vi "[ToBeTest] Continuous Complete Measurament RT.vi"() -> ()   [LabVIEW 2014]
uses:
  <vilib>/FPGAPlugInAG/sbRIO-9636/niLvFpga_Open_sbRIO-9636.vi
  <vilib>/rvi/interface/common/dynamic/niFpgaDynamicAddResources.vi
  <vilib>/FPGAPlugInAG/Dynamic/niLvFpga_Reset_Dynamic.vi
  <vilib>/Utility/error.llb/Error Cluster From Error Code.vi
  <vilib>/rvi/errors/niLvFpgaAdjustHostInterfaceError.vi
  <vilib>/rvi/interface/common/niFpgaWaitOnOcc.vi
  <vilib>/FPGAPlugInAG/Dynamic/niLvFpga_Run_Dynamic.vi
  <vilib>/FPGAPlugInAG/Dynamic/niLvFpga_Abort_Dynamic.vi
  <vilib>/FPGAPlugInAG/Dynamic/niLvFpga_Close_Dynamic.vi
  <vilib>/rvi/interface/nirviOpenFPGA/nirviOpenFPGA.xnode
  FPGA Bitfiles/LaserDistanceSen_FPGATarget_N-ParametricDoub_TAOECtWtfmQ.lvbitx
  FPGA Target/Test VIs/N-Parametric Double FFT Mesurament (MAX BIN DETECT) Test.vi
  FPGA Bitfiles/LaserDistanceSen_FPGATarget_N-ParametricDoub_oZd6Q4K0Aos.lvbitx
  FPGA Target/Test VIs/N-Parametric Double FFT Mesurament (MAX BIN DETECT) SLOW Test.vi
  <vilib>/rvi/interface/nirviMethod/nirviMethod.xnode
  <vilib>/rvi/interface/nirviReadWriteControl/nirviReadWriteControl.xnode
  <vilib>/rvi/interface/nirviCloseFPGA/nirviCloseFPGA.xnode
  <vilib>/rvi/errors/niLvFpgaMergeErrorWithErrorCode.vi
  <vilib>/rvi/interface/Simulation/niFpgaSimulationCallBeginRW.vi
  NiFpgaLv.dll
  <vilib>/Analysis/NI_AALBase.lvlib
  <vilib>/FPGAPlugInAG/Dynamic/niLvFpga_ConfigureFifo_Dynamic.vi
  <vilib>/FPGAPlugInAG/Dynamic/niLvFpga_StartFifo_Dynamic.vi
  <vilib>/FPGAPlugInAG/Dynamic/niLvFpga_ReadFifo_Dynamic.vi
panel:
  out "Rel Std Dev":dbl(graph)
  out "Mean distance":dbl(graph)
  in  "init scart":i32=2000
  out "End":bool
  in  "Fixed Measure?":bool
  in  "#signal":i32=3000
  out "Distance moving Rel Standard Deviation":dbl format="%0.7f"
  out "Distance moving mean":dbl format="%0.7f"
  in  "stop":bool
  # "Mean"
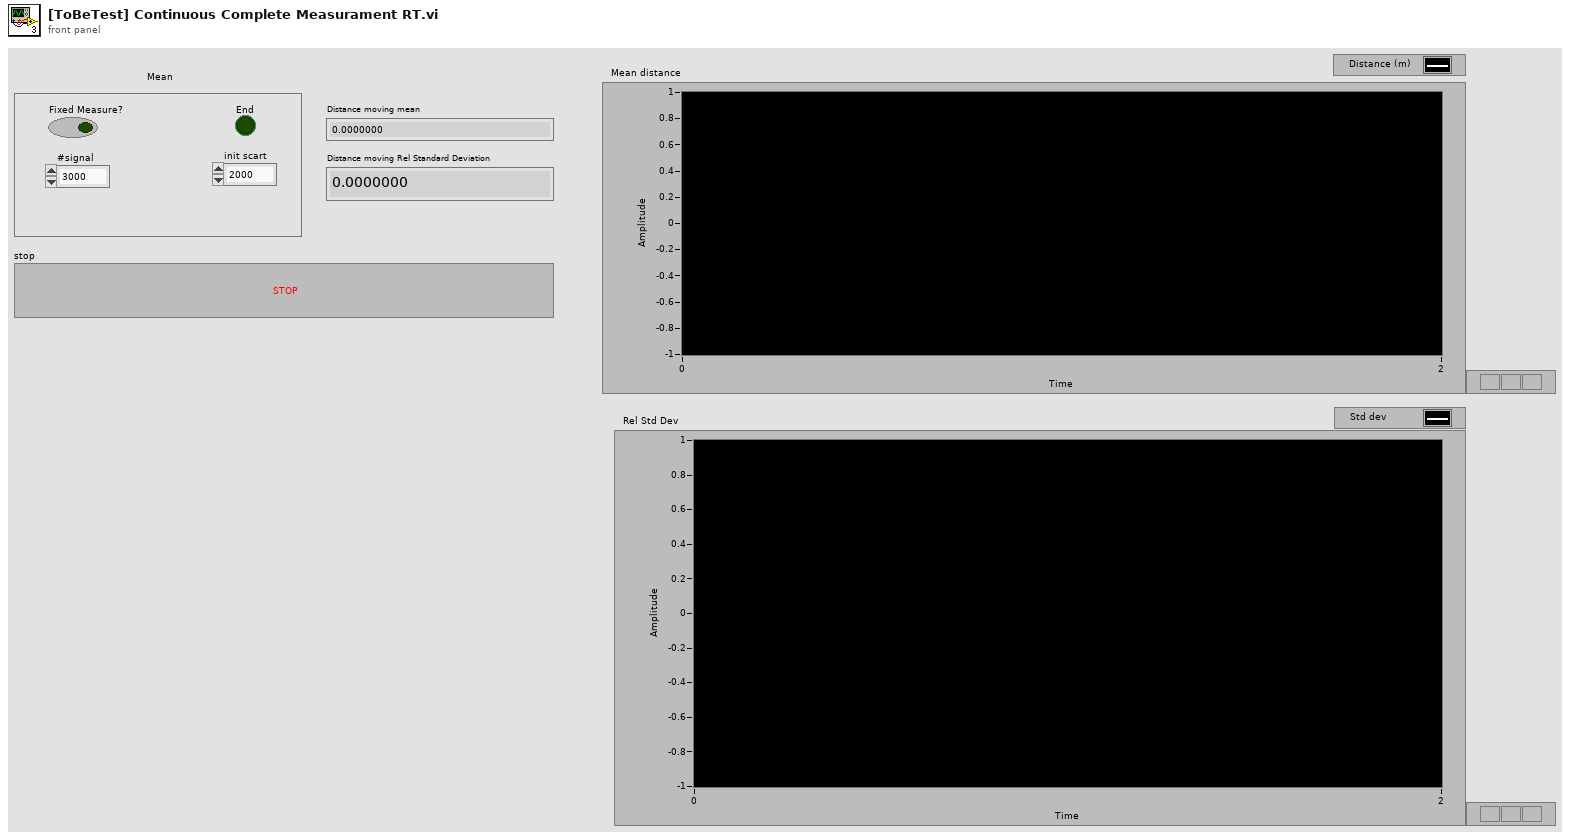
[diagram p1: front panel]
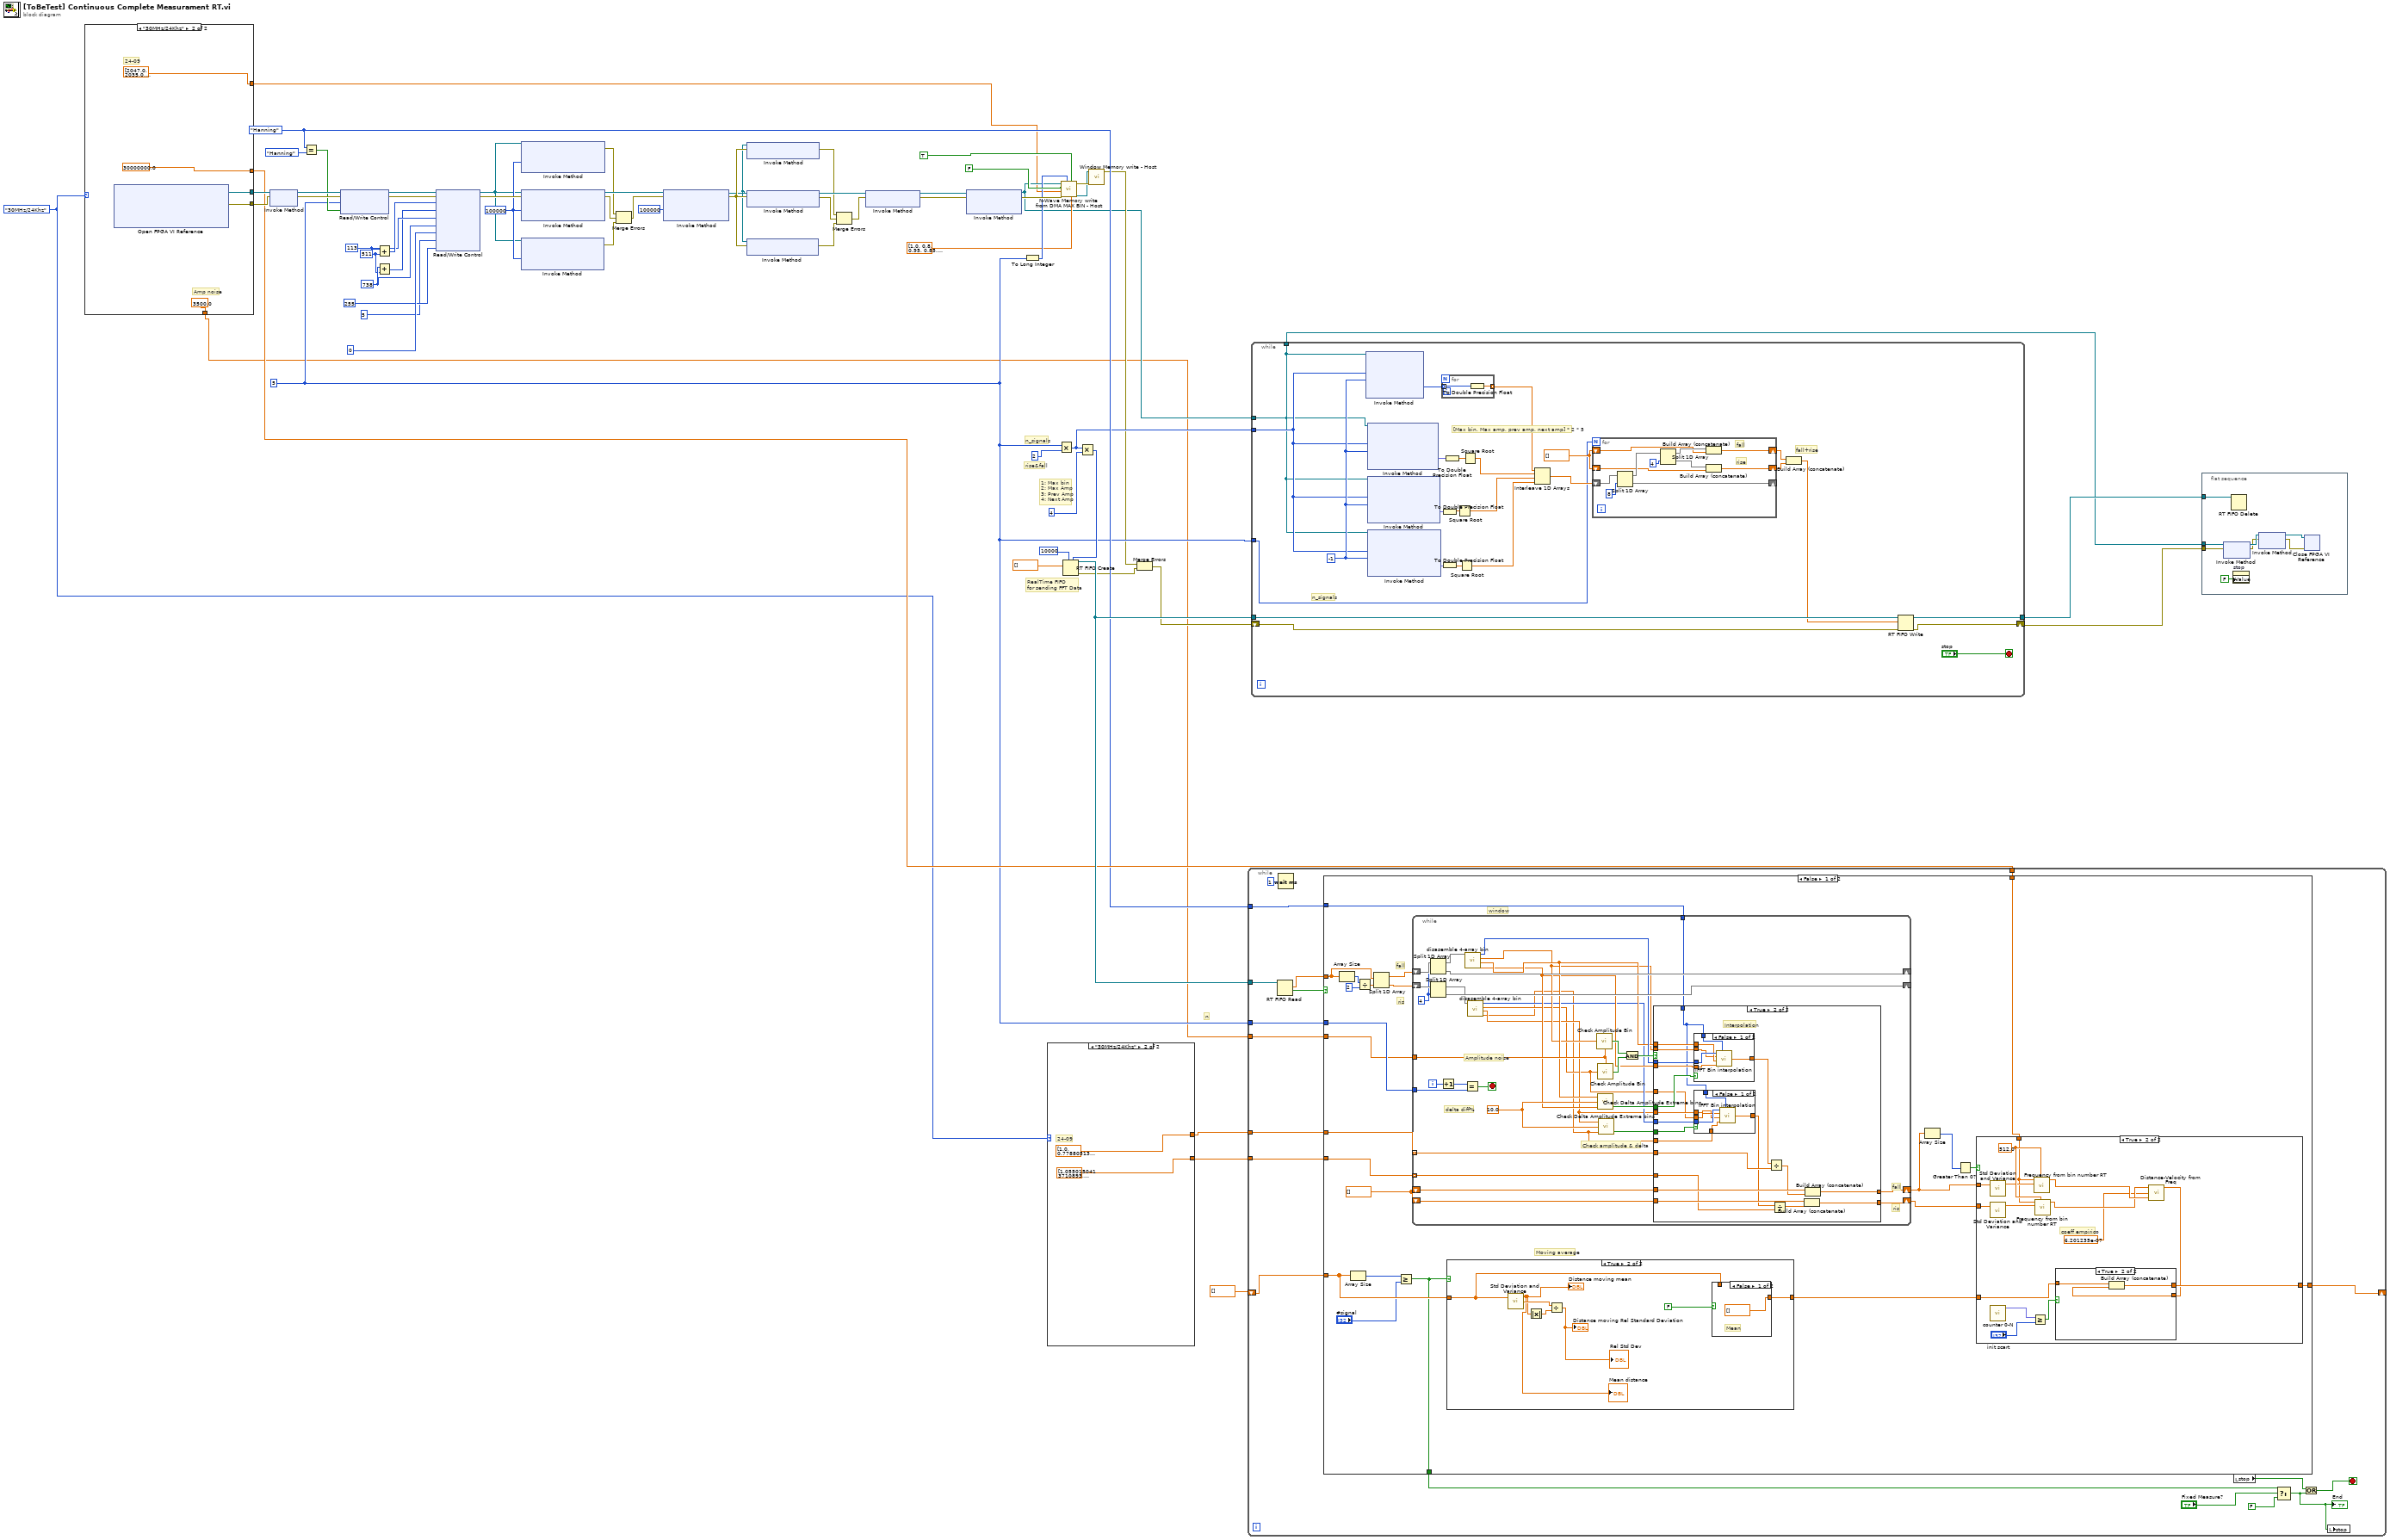
[diagram p0: block diagram]
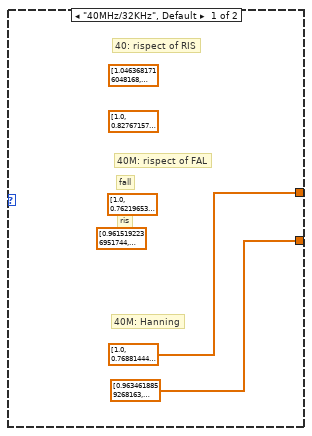
[diagram p2: hidden frame]
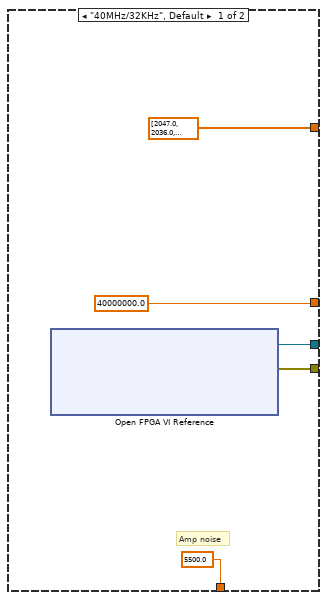
[diagram p3: hidden frame]
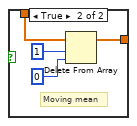
[diagram p5: hidden frame]
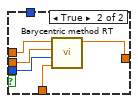
[diagram p9: hidden frame]
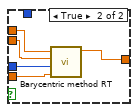
[diagram p10: hidden frame]
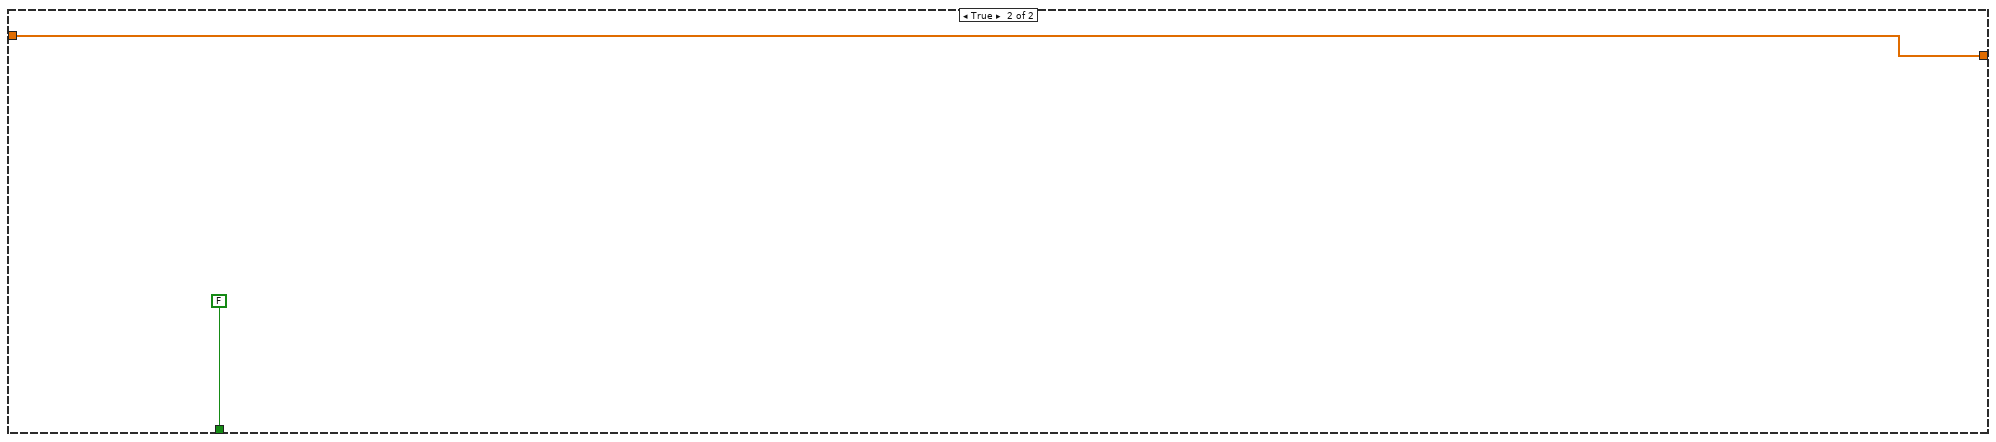
[diagram p11: hidden frame]
diagram:
  w43 = enum16{"None", "Hanning"}."Hanning" ("Windowing")
  w61 = u32 738 ("lower limit 2")
  w63 = u32 113 ("lower limit 1")
  w20 = u32 5 ("#Signals")
  w1 = enum32{"40MHz/32KHz", "30MHz/24Khz"}."30MHz/24Khz" ("Sample /Modulation Frequency")
  w38 = u32 100000 ("Requested Depth")
  w60 = u32 511 ("y")
  # "n_signals"
  # "rise&fall"
  # "1: Max bin\n2: Max Amp\n3: Prev Amp\n4: Next Amp"
  # "n"
  # "RealTime FIFO \nfor sending FFT Data"
  n1 = case shown="\"30MHz/24Khz\"" w1 {
    tunnel: [w69 w74] -> w55
    tunnel: [w68 w73] -> w54
    tunnel: [40000000.0 30000000.0] -> w46
    tunnel: [5500.0 ("Threshold Amp") 3500.0 ("Threshold Amp")] -> w3
    tunnel: [dbl[] [2047.0, 2036.0, 2024.0, 2013.0, 2002.0, 1990.0, 1979.0, 1968.0, 1956.0, 1945.0, 1934.0, 1923.0, 1912.0, 1900.0, 1889.0, 1878.0, 1867.0, 1856.0, 1845.0, 1833.0, 1822.0, 1811.0, 1800.0, 1789.0, 1778.0, 1767.0, 1756.0, 1745.0, 1734.0, 1723.0, 1712.0, 1702.0, 1691.0, 1680.0, 1669.0, 1658.0, 1647.0, 1636.0, 1626.0, 1615.0, 1604.0, 1593.0, 1583.0, 1572.0, 1561.0, 1550.0, 1540.0, 1529.0, 1518.0, 1508.0, 1497.0, 1487.0, 1476.0, 1465.0, 1455.0, 1444.0, 1434.0, 1423.0, 1413.0, 1402.0, 1392.0, 1381.0, 1371.0, 1360.0, 1350.0, 1340.0, 1329.0, 1319.0, 1309.0, 1298.0, 1288.0, 1278.0, 1267.0, 1257.0, 1247.0, 1237.0, 1226.0, 1216.0, 1206.0, 1196.0, 1186.0, 1176.0, 1165.0, 1155.0, 1145.0, 1135.0, 1125.0, 1115.0, 1105.0, 1095.0, 1085.0, 1075.0, 1065.0, 1055.0, 1045.0, 1035.0, 1025.0, 1015.0, 1006.0, 996.0, 986.0, 976.0, 966.0, 956.0, 947.0, 937.0, 927.0, 917.0, 908.0, 898.0, 888.0, 879.0, 869.0, 859.0, 850.0, 837.0, 826.0, 816.0, 804.0, 796.0, 788.0, 778.0, 769.0, 758.0, 750.0, 743.0, 733.0, 724.0, 717.0, 709.0, 701.0, 693.0, 686.0, 677.0, 669.0, 661.0, 653.0, 645.0, 638.0, 630.0, 622.0, 615.0, 607.0, 599.0, 592.0, 583.0, 576.0, 569.0, 561.0, 554.0, 547.0, 539.0, 532.0, 525.0, 518.0, 509.0, 501.0, 492.0, 486.0, 478.0, 471.0, 463.0, 456.0, 450.0, 442.0, 435.0, 429.0, 421.0, 415.0, 408.0, 401.0, 394.0, 388.0, 381.0, 375.0, 368.0, 361.0, 355.0, 349.0, 342.0, 336.0, 330.0, 323.0, 317.0, 311.0, 304.0, 298.0, 292.0, 286.0, 279.0, 273.0, 267.0, 261.0, 255.0, 249.0, 242.0, 236.0, 230.0, 224.0, 218.0, 212.0, 206.0, 200.0, 194.0, 187.0, 181.0, 175.0, 169.0, 163.0, 157.0, 150.0, 144.0, 138.0, 132.0, 125.0, 119.0, 113.0, 107.0, 101.0, 95.0, 88.0, 82.0, 77.0, 71.0, 65.0, 59.0, 53.0, 47.0, 41.0, 35.0, 29.0, 23.0, 18.0, 11.0, 6.0, 0.0, -6.0, -12.0, -18.0, -23.0, -29.0, -35.0, -41.0, -47.0, -52.0, -58.0, -64.0, -69.0, -75.0, -81.0, -87.0, -92.0, -98.0, -104.0, -109.0, -115.0, -121.0, -126.0, -132.0, -138.0, -144.0, -149.0, -155.0, -161.0, -166.0, -172.0, -177.0, -183.0, -189.0, -194.0, -200.0, -205.0, -211.0, -216.0, -222.0, -227.0, -233.0, -238.0, -244.0, -249.0, -255.0, -260.0, -266.0, -271.0, -277.0, -283.0, -288.0, -294.0, -299.0, -304.0, -310.0, -315.0, -321.0, -326.0, -331.0, -337.0, -342.0, -348.0, -353.0, -358.0, -364.0, -369.0, -375.0, -380.0, -385.0, -391.0, -396.0, -402.0, -407.0, -413.0, -418.0, -423.0, -429.0, -434.0, -439.0, -445.0, -450.0, -456.0, -461.0, -466.0, -472.0, -477.0, -483.0, -488.0, -493.0, -499.0, -504.0, -510.0, -515.0, -520.0, -526.0, -531.0, -537.0, -542.0, -548.0, -553.0, -558.0, -564.0, -569.0, -574.0, -580.0, -585.0, -590.0, -596.0, -601.0, -606.0, -612.0, -617.0, -622.0, -628.0, -633.0, -638.0, -644.0, -649.0, -654.0, -660.0, -665.0, -670.0, -676.0, -681.0, -686.0, -692.0, -697.0, -702.0, -708.0, -713.0, -718.0, -723.0, -729.0, -734.0, -739.0, -744.0, -750.0, -755.0, -760.0, -765.0, -771.0, -776.0, -781.0, -786.0, -792.0, -797.0, -802.0, -807.0, -812.0, -818.0, -823.0, -828.0, -833.0, -839.0, -844.0, -849.0, -854.0, -859.0, -865.0, -870.0, -875.0, -880.0, -885.0, -891.0, -896.0, -901.0, -906.0, -911.0, -916.0, -922.0, -927.0, -932.0, -937.0, -943.0, -948.0, -953.0, -958.0, -963.0, -969.0, -974.0, -979.0, -984.0, -989.0, -995.0, -1000.0, -1005.0, -1010.0, -1015.0, -1021.0, -1026.0, -1031.0, -1036.0, -1041.0, -1047.0, -1052.0, -1057.0, -1062.0, -1067.0, -1073.0, -1078.0, -1083.0, -1088.0, -1093.0, -1099.0, -1104.0, -1109.0, -1114.0, -1119.0, -1124.0, -1130.0, -1135.0, -1140.0, -1145.0, -1150.0, -1156.0, -1161.0, -1166.0, -1171.0, -1176.0, -1182.0, -1187.0, -1192.0, -1197.0, -1202.0, -1207.0, -1213.0, -1218.0, -1223.0, -1228.0, -1233.0, -1238.0, -1244.0, -1249.0, -1254.0, -1259.0, -1264.0, -1269.0, -1275.0, -1280.0, -1285.0, -1290.0, -1295.0, -1300.0, -1305.0, -1311.0, -1316.0, -1321.0, -1326.0, -1331.0, -1336.0, -1342.0, -1347.0, -1352.0, -1357.0, -1362.0, -1367.0, -1372.0, -1378.0, -1383.0, -1388.0, -1393.0, -1398.0, -1403.0, -1408.0, -1414.0, -1419.0, -1424.0, -1429.0, -1434.0, -1439.0, -1444.0, -1450.0, -1455.0, -1460.0, -1465.0, -1470.0, -1475.0, -1480.0, -1486.0, -1491.0, -1496.0, -1501.0, -1506.0, -1511.0, -1516.0, -1522.0, -1527.0, -1532.0, -1537.0, -1542.0, -1547.0, -1552.0, -1558.0, -1563.0, -1568.0, -1573.0, -1578.0, -1583.0, -1588.0, -1593.0, -1599.0, -1604.0, -1609.0, -1614.0, -1619.0, -1624.0, -1629.0, -1634.0, -1640.0, -1645.0, -1650.0, -1655.0, -1660.0, -1665.0, -1670.0, -1675.0, -1681.0, -1686.0, -1691.0, -1696.0, -1701.0, -1706.0, -1711.0, -1716.0, -1722.0, -1727.0, -1732.0, -1737.0, -1742.0, -1747.0, -1752.0, -1757.0, -1762.0, -1768.0, -1773.0, -1778.0, -1783.0, -1788.0, -1793.0, -1798.0, -1803.0, -1808.0, -1814.0, -1819.0, -1824.0, -1829.0, -1834.0, -1839.0, -1844.0, -1849.0, -1854.0, -1859.0, -1865.0, -1870.0, -1875.0, -1880.0, -1885.0, -1890.0, -1895.0, -1900.0, -1905.0, -1911.0, -1916.0, -1921.0, -1926.0, -1931.0, -1936.0, -1941.0, -1946.0, -1951.0, -1956.0, -1961.0, -1967.0, -1972.0, -1977.0, -1982.0, -1987.0, -1992.0, -1997.0, -2002.0, -2007.0, -2012.0, -2017.0, -2023.0, -2028.0, -2033.0, -2038.0, -2043.0, -2048.0, -2047.0, -2034.0, -2021.0, -2009.0, -1996.0, -1983.0, -1970.0, -1957.0, -1945.0, -1932.0, -1919.0, -1907.0, -1894.0, -1881.0, -1869.0, -1856.0, -1844.0, -1831.0, -1819.0, -1806.0, -1794.0, -1781.0, -1769.0, -1757.0, -1744.0, -1732.0, -1719.0, -1707.0, -1695.0, -1682.0, -1670.0, -1658.0, -1646.0, -1634.0, -1621.0, -1609.0, -1597.0, -1585.0, -1573.0, -1561.0, -1549.0, -1537.0, -1525.0, -1513.0, -1501.0, -1489.0, -1477.0, -1465.0, -1453.0, -1441.0, -1429.0, -1417.0, -1405.0, -1394.0, -1382.0, -1370.0, -1358.0, -1347.0, -1335.0, -1323.0, -1312.0, -1300.0, -1288.0, -1277.0, -1265.0, -1254.0, -1242.0, -1231.0, -1219.0, -1208.0, -1196.0, -1185.0, -1173.0, -1162.0, -1150.0, -1139.0, -1128.0, -1116.0, -1105.0, -1094.0, -1083.0, -1071.0, -1060.0, -1049.0, -1038.0, -1027.0, -1015.0, -1004.0, -993.0, -982.0, -971.0, -960.0, -949.0, -938.0, -927.0, -916.0, -905.0, -894.0, -883.0, -873.0, -862.0, -851.0, -840.0, -829.0, -819.0, -808.0, -797.0, -786.0, -776.0, -765.0, -754.0, -744.0, -733.0, -722.0, -712.0, -697.0, -685.0, -674.0, -661.0, -652.0, -643.0, -632.0, -622.0, -610.0, -602.0, -594.0, -583.0, -574.0, -566.0, -558.0, -550.0, -542.0, -534.0, -525.0, -516.0, -507.0, -499.0, -491.0, -483.0, -475.0, -467.0, -459.0, -451.0, -443.0, -435.0, -426.0, -419.0, -411.0, -404.0, -396.0, -388.0, -381.0, -373.0, -366.0, -359.0, -349.0, -341.0, -331.0, -325.0, -317.0, -309.0, -301.0, -295.0, -288.0, -280.0, -273.0, -266.0, -259.0, -252.0, -246.0, -239.0, -231.0, -225.0, -219.0, -212.0, -205.0, -199.0, -192.0, -186.0, -180.0, -173.0, -167.0, -161.0, -155.0, -148.0, -142.0, -136.0, -130.0, -124.0, -118.0, -112.0, -106.0, -100.0, -94.0, -88.0, -82.0, -76.0, -70.0, -64.0, -58.0, -52.0, -46.0, -40.0, -34.0, -28.0, -21.0, -15.0, -9.0, -3.0, 2.0, 9.0, 15.0, 21.0, 27.0, 33.0, 39.0, 45.0, 51.0, 57.0, 63.0, 69.0, 75.0, 81.0, 86.0, 92.0, 98.0, 103.0, 110.0, 116.0, 121.0, 127.0, 133.0, 138.0, 144.0, 149.0, 155.0, 161.0, 166.0, 172.0, 177.0, 183.0, 189.0, 194.0, 200.0, 205.0, 211.0, 216.0, 221.0, 227.0, 232.0, 238.0, 243.0, 249.0, 254.0, 259.0, 265.0, 270.0, 276.0, 281.0, 286.0, 292.0, 297.0, 303.0, 308.0, 314.0, 319.0, 324.0, 329.0, 335.0, 340.0, 345.0, 351.0, 356.0, 361.0, 366.0, 371.0, 377.0, 382.0, 387.0, 392.0, 397.0, 403.0, 408.0, 413.0, 418.0, 423.0, 429.0, 434.0, 439.0, 444.0, 449.0, 454.0, 459.0, 464.0, 469.0, 474.0, 479.0, 484.0, 489.0, 494.0, 499.0, 504.0, 509.0, 514.0, 520.0, 525.0, 530.0, 535.0, 540.0, 545.0, 550.0, 555.0, 560.0, 565.0, 570.0, 575.0, 580.0, 585.0, 590.0, 595.0, 600.0, 605.0, 610.0, 615.0, 620.0, 625.0, 630.0, 636.0, 641.0, 646.0, 651.0, 656.0, 661.0, 666.0, 671.0, 676.0, 681.0, 686.0, 691.0, 696.0, 701.0, 706.0, 711.0, 716.0, 721.0, 726.0, 731.0, 736.0, 741.0, 746.0, 751.0, 756.0, 761.0, 765.0, 770.0, 775.0, 780.0, 785.0, 790.0, 795.0, 800.0, 805.0, 810.0, 815.0, 820.0, 825.0, 829.0, 834.0, 839.0, 844.0, 849.0, 854.0, 859.0, 864.0, 868.0, 873.0, 878.0, 883.0, 888.0, 893.0, 897.0, 902.0, 907.0, 912.0, 917.0, 921.0, 926.0, 931.0, 936.0, 941.0, 945.0, 950.0, 955.0, 960.0, 965.0, 969.0, 974.0, 979.0, 984.0, 988.0, 993.0, 998.0, 1003.0, 1007.0, 1012.0, 1017.0, 1022.0, 1027.0, 1031.0, 1036.0, 1041.0, 1046.0, 1051.0, 1055.0, 1060.0, 1065.0, 1070.0, 1075.0, 1079.0, 1084.0, 1089.0, 1094.0, 1098.0, 1103.0, 1108.0, 1113.0, 1118.0, 1122.0, 1127.0, 1132.0, 1137.0, 1141.0, 1146.0, 1151.0, 1156.0, 1161.0, 1165.0, 1170.0, 1175.0, 1180.0, 1184.0, 1189.0, 1194.0, 1199.0, 1204.0, 1208.0, 1213.0, 1218.0, 1223.0, 1227.0, 1232.0, 1237.0, 1242.0, 1246.0, 1251.0, 1256.0, 1261.0, 1265.0, 1270.0, 1275.0, 1280.0, 1284.0, 1289.0, 1294.0, 1299.0, 1303.0, 1308.0, 1313.0, 1318.0, 1322.0, 1327.0, 1332.0, 1336.0, 1341.0, 1346.0, 1351.0, 1355.0, 1360.0, 1365.0, 1370.0, 1374.0, 1379.0, 1384.0, 1388.0, 1393.0, 1398.0, 1403.0, 1407.0, 1412.0, 1417.0, 1421.0, 1426.0, 1431.0, 1436.0, 1440.0, 1445.0, 1450.0, 1454.0, 1459.0, 1464.0, 1469.0, 1473.0, 1478.0, 1483.0, 1487.0, 1492.0, 1497.0, 1502.0, 1506.0, 1511.0, 1516.0, 1520.0, 1525.0, 1530.0, 1535.0, 1539.0, 1544.0, 1549.0, 1553.0, 1558.0, 1563.0, 1567.0, 1572.0, 1577.0, 1582.0, 1586.0, 1591.0, 1596.0, 1600.0, 1605.0, 1610.0, 1614.0, 1619.0, 1624.0, 1628.0, 1633.0, 1638.0, 1643.0, 1647.0, 1652.0, 1657.0, 1661.0, 1666.0, 1671.0, 1675.0, 1680.0, 1685.0, 1689.0, 1694.0, 1699.0, 1703.0, 1708.0, 1713.0, 1717.0, 1722.0, 1727.0, 1731.0, 1736.0, 1741.0, 1746.0, 1750.0, 1755.0, 1760.0, 1764.0, 1769.0, 1774.0, 1778.0, 1783.0, 1788.0, 1792.0, 1797.0, 1802.0, 1806.0, 1811.0, 1816.0, 1820.0, 1825.0, 1830.0, 1834.0, 1839.0, 1844.0, 1848.0, 1853.0, 1858.0, 1862.0, 1867.0, 1871.0, 1876.0, 1881.0, 1885.0, 1890.0, 1895.0, 1899.0, 1904.0, 1909.0, 1913.0, 1918.0, 1923.0, 1927.0, 1932.0, 1937.0, 1941.0, 1946.0, 1951.0, 1955.0, 1960.0, 1965.0, 1969.0, 1974.0, 1978.0, 1983.0, 1988.0, 1992.0, 1997.0, 2002.0, 2006.0, 2011.0, 2016.0, 2020.0, 2025.0, 2029.0, 2034.0, 2039.0, 2043.0, 2048.0] ("Complete SkewTri") dbl[] [2047.0, 2035.0, 2022.0, 2010.0, 1997.0, 1985.0, 1972.0, 1960.0, 1948.0, 1935.0, 1923.0, 1911.0, 1899.0, 1886.0, 1874.0, 1862.0, 1850.0, 1838.0, 1825.0, 1813.0, 1801.0, 1789.0, 1777.0, 1765.0, 1753.0, 1741.0, 1729.0, 1717.0, 1705.0, 1693.0, 1681.0, 1669.0, 1657.0, 1645.0, 1634.0, 1622.0, 1610.0, 1598.0, 1586.0, 1575.0, 1563.0, 1551.0, 1540.0, 1528.0, 1516.0, 1505.0, 1493.0, 1481.0, 1470.0, 1458.0, 1447.0, 1435.0, 1424.0, 1412.0, 1401.0, 1389.0, 1378.0, 1366.0, 1355.0, 1344.0, 1332.0, 1321.0, 1310.0, 1298.0, 1287.0, 1276.0, 1265.0, 1253.0, 1242.0, 1231.0, 1220.0, 1209.0, 1198.0, 1186.0, 1175.0, 1164.0, 1153.0, 1142.0, 1131.0, 1120.0, 1109.0, 1098.0, 1087.0, 1076.0, 1065.0, 1055.0, 1044.0, 1033.0, 1022.0, 1011.0, 1000.0, 990.0, 979.0, 968.0, 958.0, 947.0, 936.0, 926.0, 915.0, 904.0, 894.0, 883.0, 873.0, 862.0, 852.0, 841.0, 831.0, 820.0, 810.0, 799.0, 789.0, 778.0, 768.0, 758.0, 747.0, 738.0, 727.0, 719.0, 712.0, 706.0, 700.0, 693.0, 687.0, 680.0, 674.0, 668.0, 661.0, 655.0, 648.0, 642.0, 636.0, 629.0, 623.0, 617.0, 610.0, 604.0, 598.0, 591.0, 584.0, 577.0, 569.0, 560.0, 552.0, 545.0, 538.0, 531.0, 525.0, 519.0, 512.0, 506.0, 500.0, 494.0, 488.0, 482.0, 476.0, 470.0, 464.0, 458.0, 452.0, 446.0, 436.0, 430.0, 424.0, 418.0, 412.0, 406.0, 400.0, 394.0, 388.0, 382.0, 376.0, 370.0, 364.0, 358.0, 352.0, 346.0, 338.0, 332.0, 325.0, 319.0, 313.0, 307.0, 301.0, 295.0, 290.0, 284.0, 278.0, 272.0, 267.0, 261.0, 255.0, 249.0, 244.0, 238.0, 232.0, 227.0, 221.0, 215.0, 209.0, 204.0, 198.0, 192.0, 187.0, 181.0, 175.0, 170.0, 164.0, 158.0, 153.0, 147.0, 141.0, 136.0, 130.0, 124.0, 119.0, 113.0, 108.0, 102.0, 96.0, 91.0, 85.0, 79.0, 74.0, 68.0, 62.0, 57.0, 51.0, 45.0, 39.0, 34.0, 28.0, 22.0, 16.0, 11.0, 5.0, 0.0, -6.0, -11.0, -17.0, -22.0, -28.0, -33.0, -39.0, -44.0, -50.0, -55.0, -61.0, -66.0, -72.0, -77.0, -83.0, -88.0, -94.0, -99.0, -105.0, -110.0, -116.0, -121.0, -127.0, -132.0, -137.0, -143.0, -148.0, -154.0, -159.0, -165.0, -170.0, -176.0, -181.0, -186.0, -192.0, -197.0, -203.0, -208.0, -214.0, -219.0, -224.0, -230.0, -235.0, -241.0, -246.0, -251.0, -257.0, -262.0, -268.0, -273.0, -278.0, -284.0, -289.0, -295.0, -300.0, -305.0, -311.0, -316.0, -321.0, -327.0, -332.0, -337.0, -343.0, -348.0, -354.0, -359.0, -364.0, -370.0, -375.0, -380.0, -386.0, -391.0, -397.0, -402.0, -407.0, -413.0, -418.0, -423.0, -429.0, -434.0, -439.0, -445.0, -450.0, -455.0, -461.0, -466.0, -471.0, -477.0, -482.0, -487.0, -493.0, -498.0, -503.0, -509.0, -514.0, -519.0, -525.0, -530.0, -535.0, -540.0, -546.0, -551.0, -556.0, -562.0, -567.0, -572.0, -578.0, -583.0, -588.0, -593.0, -599.0, -604.0, -609.0, -615.0, -620.0, -625.0, -630.0, -636.0, -641.0, -646.0, -651.0, -657.0, -662.0, -667.0, -673.0, -678.0, -683.0, -688.0, -694.0, -699.0, -704.0, -709.0, -715.0, -720.0, -725.0, -730.0, -736.0, -741.0, -746.0, -751.0, -757.0, -762.0, -767.0, -772.0, -778.0, -783.0, -788.0, -793.0, -799.0, -804.0, -809.0, -814.0, -820.0, -825.0, -830.0, -835.0, -841.0, -846.0, -851.0, -856.0, -862.0, -867.0, -872.0, -877.0, -883.0, -888.0, -893.0, -898.0, -903.0, -909.0, -914.0, -919.0, -924.0, -930.0, -935.0, -940.0, -945.0, -951.0, -956.0, -961.0, -966.0, -971.0, -977.0, -982.0, -987.0, -992.0, -998.0, -1003.0, -1008.0, -1013.0, -1018.0, -1024.0, -1029.0, -1034.0, -1039.0, -1045.0, -1050.0, -1055.0, -1060.0, -1065.0, -1071.0, -1076.0, -1081.0, -1086.0, -1092.0, -1097.0, -1102.0, -1107.0, -1112.0, -1118.0, -1123.0, -1128.0, -1133.0, -1138.0, -1144.0, -1149.0, -1154.0, -1159.0, -1165.0, -1170.0, -1175.0, -1180.0, -1185.0, -1191.0, -1196.0, -1201.0, -1206.0, -1211.0, -1217.0, -1222.0, -1227.0, -1232.0, -1237.0, -1243.0, -1248.0, -1253.0, -1258.0, -1263.0, -1269.0, -1274.0, -1279.0, -1284.0, -1289.0, -1295.0, -1300.0, -1305.0, -1310.0, -1315.0, -1321.0, -1326.0, -1331.0, -1336.0, -1341.0, -1347.0, -1352.0, -1357.0, -1362.0, -1367.0, -1373.0, -1378.0, -1383.0, -1388.0, -1393.0, -1399.0, -1404.0, -1409.0, -1414.0, -1419.0, -1425.0, -1430.0, -1435.0, -1440.0, -1445.0, -1450.0, -1456.0, -1461.0, -1466.0, -1471.0, -1476.0, -1482.0, -1487.0, -1492.0, -1497.0, -1502.0, -1508.0, -1513.0, -1518.0, -1523.0, -1528.0, -1534.0, -1539.0, -1544.0, -1549.0, -1554.0, -1560.0, -1565.0, -1570.0, -1575.0, -1580.0, -1586.0, -1591.0, -1596.0, -1601.0, -1606.0, -1612.0, -1617.0, -1622.0, -1627.0, -1632.0, -1637.0, -1643.0, -1648.0, -1653.0, -1658.0, -1663.0, -1669.0, -1674.0, -1679.0, -1684.0, -1689.0, -1695.0, -1700.0, -1705.0, -1710.0, -1715.0, -1721.0, -1726.0, -1731.0, -1736.0, -1741.0, -1747.0, -1752.0, -1757.0, -1762.0, -1767.0, -1773.0, -1778.0, -1783.0, -1788.0, -1793.0, -1799.0, -1804.0, -1809.0, -1814.0, -1819.0, -1825.0, -1830.0, -1835.0, -1840.0, -1845.0, -1851.0, -1856.0, -1861.0, -1866.0, -1871.0, -1876.0, -1882.0, -1887.0, -1892.0, -1897.0, -1902.0, -1908.0, -1913.0, -1918.0, -1923.0, -1928.0, -1934.0, -1939.0, -1944.0, -1949.0, -1954.0, -1960.0, -1965.0, -1970.0, -1975.0, -1980.0, -1986.0, -1991.0, -1996.0, -2001.0, -2006.0, -2012.0, -2017.0, -2022.0, -2027.0, -2032.0, -2038.0, -2043.0, -2048.0, -2047.0, -2037.0, -2027.0, -2017.0, -2007.0, -1997.0, -1987.0, -1977.0, -1967.0, -1957.0, -1947.0, -1937.0, -1927.0, -1917.0, -1907.0, -1897.0, -1888.0, -1878.0, -1868.0, -1858.0, -1848.0, -1838.0, -1828.0, -1819.0, -1809.0, -1799.0, -1789.0, -1780.0, -1770.0, -1760.0, -1750.0, -1741.0, -1731.0, -1721.0, -1712.0, -1702.0, -1692.0, -1683.0, -1673.0, -1663.0, -1654.0, -1644.0, -1635.0, -1625.0, -1615.0, -1606.0, -1596.0, -1587.0, -1577.0, -1568.0, -1558.0, -1549.0, -1539.0, -1530.0, -1520.0, -1511.0, -1501.0, -1492.0, -1483.0, -1473.0, -1464.0, -1454.0, -1445.0, -1436.0, -1426.0, -1417.0, -1408.0, -1398.0, -1389.0, -1380.0, -1371.0, -1361.0, -1352.0, -1343.0, -1334.0, -1324.0, -1315.0, -1306.0, -1297.0, -1288.0, -1278.0, -1269.0, -1260.0, -1251.0, -1242.0, -1233.0, -1224.0, -1215.0, -1205.0, -1196.0, -1187.0, -1178.0, -1169.0, -1160.0, -1151.0, -1142.0, -1133.0, -1124.0, -1115.0, -1106.0, -1097.0, -1088.0, -1080.0, -1071.0, -1062.0, -1053.0, -1044.0, -1035.0, -1026.0, -1017.0, -1009.0, -1000.0, -991.0, -982.0, -973.0, -965.0, -953.0, -944.0, -935.0, -920.0, -906.0, -889.0, -871.0, -854.0, -842.0, -834.0, -826.0, -818.0, -810.0, -802.0, -794.0, -786.0, -778.0, -770.0, -762.0, -754.0, -746.0, -739.0, -731.0, -723.0, -715.0, -707.0, -699.0, -690.0, -682.0, -672.0, -661.0, -651.0, -639.0, -627.0, -616.0, -606.0, -598.0, -591.0, -584.0, -577.0, -570.0, -563.0, -556.0, -549.0, -542.0, -535.0, -528.0, -520.0, -513.0, -506.0, -499.0, -492.0, -485.0, -478.0, -471.0, -464.0, -457.0, -451.0, -444.0, -437.0, -430.0, -423.0, -416.0, -409.0, -400.0, -390.0, -382.0, -373.0, -364.0, -356.0, -349.0, -343.0, -336.0, -330.0, -323.0, -317.0, -310.0, -304.0, -297.0, -291.0, -284.0, -278.0, -271.0, -265.0, -258.0, -252.0, -245.0, -239.0, -232.0, -226.0, -219.0, -213.0, -207.0, -200.0, -194.0, -187.0, -181.0, -175.0, -168.0, -162.0, -156.0, -149.0, -143.0, -136.0, -128.0, -121.0, -114.0, -107.0, -100.0, -93.0, -87.0, -80.0, -74.0, -68.0, -62.0, -56.0, -50.0, -44.0, -38.0, -32.0, -26.0, -20.0, -14.0, -8.0, -2.0, 5.0, 11.0, 17.0, 23.0, 29.0, 35.0, 41.0, 47.0, 53.0, 59.0, 65.0, 70.0, 76.0, 82.0, 88.0, 94.0, 100.0, 106.0, 112.0, 118.0, 124.0, 130.0, 136.0, 142.0, 148.0, 154.0, 161.0, 167.0, 174.0, 180.0, 186.0, 192.0, 198.0, 204.0, 210.0, 215.0, 221.0, 227.0, 233.0, 238.0, 244.0, 250.0, 255.0, 261.0, 267.0, 273.0, 278.0, 284.0, 290.0, 295.0, 301.0, 307.0, 312.0, 318.0, 324.0, 329.0, 335.0, 341.0, 346.0, 352.0, 358.0, 363.0, 369.0, 374.0, 380.0, 386.0, 391.0, 397.0, 402.0, 408.0, 414.0, 419.0, 425.0, 430.0, 436.0, 441.0, 447.0, 453.0, 458.0, 464.0, 470.0, 475.0, 481.0, 487.0, 493.0, 499.0, 504.0, 510.0, 516.0, 521.0, 527.0, 532.0, 538.0, 543.0, 549.0, 554.0, 560.0, 565.0, 571.0, 576.0, 582.0, 587.0, 593.0, 598.0, 604.0, 609.0, 614.0, 620.0, 625.0, 631.0, 636.0, 642.0, 647.0, 653.0, 658.0, 663.0, 669.0, 674.0, 680.0, 685.0, 691.0, 696.0, 701.0, 707.0, 712.0, 718.0, 723.0, 728.0, 734.0, 739.0, 745.0, 750.0, 755.0, 761.0, 766.0, 772.0, 777.0, 782.0, 788.0, 793.0, 798.0, 804.0, 809.0, 815.0, 820.0, 826.0, 831.0, 837.0, 842.0, 847.0, 853.0, 858.0, 863.0, 869.0, 874.0, 880.0, 885.0, 890.0, 895.0, 901.0, 906.0, 911.0, 917.0, 922.0, 927.0, 933.0, 938.0, 943.0, 948.0, 954.0, 959.0, 964.0, 970.0, 975.0, 980.0, 985.0, 991.0, 996.0, 1001.0, 1006.0, 1012.0, 1017.0, 1022.0, 1027.0, 1033.0, 1038.0, 1043.0, 1048.0, 1054.0, 1059.0, 1064.0, 1069.0, 1075.0, 1080.0, 1085.0, 1090.0, 1096.0, 1101.0, 1106.0, 1111.0, 1116.0, 1122.0, 1127.0, 1132.0, 1137.0, 1143.0, 1148.0, 1153.0, 1158.0, 1163.0, 1169.0, 1174.0, 1179.0, 1184.0, 1190.0, 1195.0, 1200.0, 1205.0, 1211.0, 1216.0, 1221.0, 1226.0, 1231.0, 1237.0, 1242.0, 1247.0, 1252.0, 1257.0, 1262.0, 1268.0, 1273.0, 1278.0, 1283.0, 1288.0, 1293.0, 1298.0, 1304.0, 1309.0, 1314.0, 1319.0, 1324.0, 1329.0, 1334.0, 1340.0, 1345.0, 1350.0, 1355.0, 1360.0, 1365.0, 1370.0, 1375.0, 1381.0, 1386.0, 1391.0, 1396.0, 1401.0, 1406.0, 1411.0, 1416.0, 1421.0, 1427.0, 1432.0, 1437.0, 1442.0, 1447.0, 1452.0, 1457.0, 1462.0, 1467.0, 1472.0, 1478.0, 1483.0, 1488.0, 1493.0, 1498.0, 1503.0, 1508.0, 1513.0, 1518.0, 1523.0, 1528.0, 1534.0, 1539.0, 1544.0, 1549.0, 1554.0, 1559.0, 1564.0, 1569.0, 1574.0, 1579.0, 1584.0, 1589.0, 1595.0, 1600.0, 1605.0, 1610.0, 1615.0, 1620.0, 1625.0, 1630.0, 1635.0, 1640.0, 1645.0, 1650.0, 1655.0, 1660.0, 1666.0, 1671.0, 1676.0, 1681.0, 1686.0, 1691.0, 1696.0, 1701.0, 1706.0, 1711.0, 1716.0, 1721.0, 1726.0, 1731.0, 1736.0, 1741.0, 1746.0, 1751.0, 1757.0, 1762.0, 1767.0, 1772.0, 1777.0, 1782.0, 1787.0, 1792.0, 1797.0, 1802.0, 1807.0, 1812.0, 1817.0, 1822.0, 1827.0, 1832.0, 1837.0, 1842.0, 1847.0, 1852.0, 1857.0, 1862.0, 1867.0, 1872.0, 1877.0, 1883.0, 1888.0, 1893.0, 1898.0, 1903.0, 1908.0, 1913.0, 1918.0, 1923.0, 1928.0, 1933.0, 1938.0, 1943.0, 1948.0, 1953.0, 1958.0, 1963.0, 1968.0, 1973.0, 1978.0, 1983.0, 1988.0, 1993.0, 1998.0, 2003.0, 2008.0, 2013.0, 2018.0, 2023.0, 2028.0, 2033.0, 2038.0, 2043.0, 2048.0] ("appended array")] -> w2
    frame "40MHz/32KHz", Default {
      # "Amp noise"
      n2 = xnode "Open FPGA VI Reference"() -> ("FPGA VI Reference Out"=w69:refnum<k20>, "error out"=w68:errorcluster)  [unwired: 2 in]
    }
    frame "30MHz/24Khz" {
      # "24-09"
      # "Amp noise"
      n3 = xnode "Open FPGA VI Reference"() -> ("FPGA VI Reference Out"=w74:refnum<k20>, "error out"=w73:errorcluster)  [unwired: 2 in]
    }
  }
  n4 = xnode "Invoke Method"("FPGA VI Reference In"=w55, "error in"=w54) -> ("FPGA VI Reference Out"=w52:refnum<k20>, "error out"=w53:errorcluster)
  n5 = Equal?(x=w43, y=enum16{"None", "Hanning"}."Hanning") -> (x = y?=w41:bool)
  n6 = xnode "Read/Write Control"("FPGA VI Reference In"=w52, "error in"=w53, "n"=w20, "Hanning window"=w41) -> ("FPGA VI Reference Out"=w51:refnum<k20>, "error out"=w50:errorcluster)
  n7 = Add(x=w63, y=w60) -> (x+y=w64:u32)
  n8 = Add(x=w61, y=w60) -> (x+y=w62:u32)
  n9 = xnode "Read/Write Control"("FPGA VI Reference In"=w51, "error in"=w50, "upper limit 1"=w64, "upper limit 2"=w62, "lower limit 1"=w63, "lower limit 2"=w61, "Latency points"=u32 0 ("Initial Latency points"), "First bin"=5 ("first bin"), "Last bin"=255 ("last bin")) -> ("FPGA VI Reference Out"=w18:refnum<k20>, "error out"=w59:errorcluster)
  n10 = xnode "Invoke Method"("FPGA VI Reference In"=w18, "Requested Depth"=w38) -> ("error out"=w37:errorcluster)  [unwired: 1 in, 2 out]
  n11 = xnode "Invoke Method"("FPGA VI Reference In"=w18, "error in"=w59, "Requested Depth"=w38) -> ("FPGA VI Reference Out"=w56:refnum<k20>, "error out"=w36:errorcluster)  [unwired: 1 out]
  n12 = xnode "Invoke Method"("FPGA VI Reference In"=w18, "Requested Depth"=w38) -> ("error out"=w35:errorcluster)  [unwired: 1 in, 2 out]
  n13 = Merge Errors(w37, w36, w35) -> (w34:errorcluster)
  n14 = xnode "Invoke Method"("FPGA VI Reference In"=w56, "error in"=w34, "Requested Depth"=u32 100000) -> ("FPGA VI Reference Out"=w26:refnum<k20>, "error out"=w27:errorcluster)  [unwired: 1 out]
  n15 = xnode "Invoke Method"("FPGA VI Reference In"=w26, "error in"=w27) -> ("error out"=w25:errorcluster)  [unwired: 1 out]
  n16 = xnode "Invoke Method"("FPGA VI Reference In"=w26, "error in"=w27) -> ("FPGA VI Reference Out"=w30:refnum<k20>, "error out"=w31:errorcluster)
  n17 = xnode "Invoke Method"("FPGA VI Reference In"=w26, "error in"=w27) -> ("error out"=w32:errorcluster)  [unwired: 1 out]
  n18 = Merge Errors(w25, w31, w32) -> (w33:errorcluster)
  n19 = xnode "Invoke Method"("FPGA VI Reference In"=w30, "error in"=w33) -> ("FPGA VI Reference Out"=w29:refnum<k20>, "error out"=w28:errorcluster)
  n20 = xnode "Invoke Method"("FPGA VI Reference In"=w29, "error in"=w28) -> ("FPGA VI Reference Out"=w4:refnum<k20>, "error out"=w10:errorcluster)  [unwired: 1 in]
  n21 = To Long Integer(number=w20) -> (32bit integer=w7:i32)
  n22 = case shown="\"30MHz/24Khz\"" w1 {
    tunnel: [dbl[] [1.0, 0.7688144425878637, 0.960709657195022, 0.8322860112544478, 0.9000054001812109] ("mean factor 1") dbl[] [1.0, 0.7788051374952276, 0.9586568902543302, 0.8395566206470091, 0.903068410955916] ("mean factor 1")] -> w45
    tunnel: [dbl[] [0.9634618859268163, 0.8014672128927146, 0.9212223217673626, 0.8422741314179902, 0.8798034158007506] ("mean factor 2") dbl[] [1.0550150413710893, 0.8807744280543515, 1.0096480344577006, 0.9233799836458207, 0.9653106595082892] ("mean factor 2")] -> w44
    frame "40MHz/32KHz", Default {
      (unwired) dbl[] [1.0, 0.8276715727566772, 0.951057672906754, 0.8699894012780883, 0.9088749122499512] ("mean factor 2")
      (unwired) dbl[] [1.0463681716048168, 0.7798670577740541, 0.9941516729466621, 0.8518960261002109, 0.9344668620862013] ("mean factor 1")
      (unwired) dbl[] [0.9615192236951744, 0.7991689735453839, 0.9195906148777597, 0.8398501694296071, 0.878805719221393] ("mean factor 2")
      (unwired) dbl[] [1.0, 0.7621965374978185, 0.9584394857997629, 0.8264927572637538, 0.8956014637747813] ("mean factor 1")
      # "40M: Hanning"
      # "40: rispect of RIS"
      # "40M: rispect of FAL"
      # "ris"
      # "fall"
    }
    frame "30MHz/24Khz" {
      # "24-09"
    }
  }
  n23 = Multiply(x=w20, y=u32 2 ("elements in array (1)")) -> (x*y=w21:u32)
  n24 = call "N-Wave Memory write from DMA MAX BIN - Host.vi"("Triangular Multiply Factor"=dbl[] [1.0, 0.8, 0.95, 0.85, 0.9], "Enable triangular scaling"=TRUE, "n"=w7, "error in"=w10, "Custom Triangular Signal (fal-ris)"=w2, "Triangolo dritto?"=FALSE, "FPGA VI Reference In"=w4) -> ("FPGA VI Reference Out"=w5:refnum<k20>, "error out"=w11:errorcluster)  [unwired: 2 in, 1 out]
  n25 = Multiply(x=w21, y=u32 4 ("elements in array (1)")) -> (x*y=w22:u32)
  n26 = RT FIFO Create(1:dbl[] [] ("first subarray"), 4:u32 10000 ("size (10)"), 6:w22) -> (8:w48:refnum<k33>, 11:w14:errorcluster)  [unwired: 5 in, 1 out]
  n27 = call "Window Memory write - Host.vi"("error in"=w11, "FPGA VI Reference In"=w5) -> ("error out"=w12:errorcluster)  [unwired: 7 in, 2 out]
  n28 = Merge Errors(w12, w14) -> (w13:errorcluster)
  n29 = while {
    tunnel: w48 -> [w96]
    tunnel: w43 -> [w93]
    tunnel: w20 -> [w92]
    shift-right: [w90] -> _
    shift-left: dbl[] [] ("appended array") -> [w91]
    tunnel: w46 -> [w89]
    tunnel: w45 -> [w88]
    tunnel: w44 -> [w87]
    tunnel: w3 -> [w86]
    stop <- w83 stop-if-true
    n30 = RT FIFO Read(0:w96) -> (9:w94:dbl[], 10:w95:bool)  [unwired: 3 in, 3 out]
    n31 = Wait (ms)(milliseconds to wait=u32 1) -> ()  [unwired: 1 out]
    n32 = case shown="False" w95 {
      tunnel: w94 -> [w119 _]
      tunnel: w93 -> [w118 _]
      tunnel: w92 -> [w115 _]
      tunnel: w91 -> [w108 w232]
      tunnel: [w106 w232] -> w90
      tunnel: w89 -> [w97 _]
      tunnel: w88 -> [w105 _]
      tunnel: w87 -> [w104 _]
      tunnel: w86 -> [w103 _]
      tunnel: [w99 FALSE] -> w80
      frame False {
        w114 = dbl[] [] ("appended array")
        # "Moving average"
        # "window"
        # "ris"
        # "fall"
        n33 = Array Size(array=w119) -> (size(s)=w102:i32)
        n34 = Array Size(array=w108) -> (size(s)=w109:i32)
        n35 = Divide(x=w102, y=2) -> (x/y=w100:dbl)
        n36 = Split 1D Array(array=w119, index=w100) -> (first subarray=w116:dbl[], second subarray=w117:dbl[])
        n37 = Greater Or Equal?(x=w109, y="#signal") -> (x >= y?=w99:bool)
        n38 = while {
          shift-right: [w177] -> _
          shift-left: w116 -> [w185]
          shift-right: [w178] -> _
          shift-left: w117 -> [w184]
          tunnel: w118 -> [w170]
          tunnel: w115 -> [w182]
          shift-right: [w169] -> w113
          shift-left: w114 -> [w167]
          shift-right: [w168] -> w112
          shift-left: w114 -> [w166]
          tunnel: w105 -> [w165] mode=indexing
          tunnel: w104 -> [w164] mode=indexing
          tunnel: w103 -> [w163]
          i -> [w179]
          stop <- w183 stop-if-true
          w176 = 10.0 ("Max Difference %")
          w181 = 4 ("x")
          # "delta diff%"
          # "ris"
          # "fall"
          # "Check amplitude & delta"
          # "Amplitude noise"
          n39 = Split 1D Array(array=w185, index=w181) -> (first subarray=w162:dbl[], second subarray=w177:dbl[])
          n40 = Split 1D Array(array=w184, index=w181) -> (first subarray=w161:dbl[], second subarray=w178:dbl[])
          n41 = Increment(x=w179) -> (x+1=w180:i32)
          n42 = Equal?(x=w180, y=w182) -> (x = y?=w183:bool)
          n43 = call "disasemble 4-array bin.vi"("4-Array Bin-Amp"=w162) -> ("Next Amp"=w157:dbl, "Prev amp"=w159:dbl, "Max amp"=w158:dbl, "Max bin"=w160:i32)  [unwired: 7 in]
          n44 = call "disasemble 4-array bin.vi"("4-Array Bin-Amp"=w161) -> ("Next Amp"=w153:dbl, "Prev amp"=w155:dbl, "Max amp"=w154:dbl, "Max bin"=w156:i32)  [unwired: 7 in]
          n45 = call "Check Amplitude Bin.vi"("Threshold Amp"=w163, "Max Amp"=w158) -> ("Check Amp Ok?"=w175:bool)  [unwired: 2 in]
          n46 = call "Check Amplitude Bin.vi"("Threshold Amp"=w163, "Max Amp"=w154) -> ("Check Amp Ok?"=w174:bool)  [unwired: 2 in]
          n47 = call "Check Delta Amplitude Extreme bins.vi"("Succ Max Amp"=w157, "Max Difference %"=w176, "Prev Max Amp"=w159) -> ("Check Delta Amp Ok?"=w172:bool)  [unwired: 1 in, 1 out]
          n48 = call "Check Delta Amplitude Extreme bins.vi"("Succ Max Amp"=w153, "Max Difference %"=w176, "Prev Max Amp"=w155) -> ("Check Delta Amp Ok?"=w171:bool)  [unwired: 1 in, 1 out]
          n49 = And(x=w175, y=w174) -> (x .and. y?=w173:bool)
          n50 = case shown="True" w173 {
            tunnel: w172 -> [_ w208]
            tunnel: w171 -> [_ w207]
            tunnel: w155 -> [_ w206]
            tunnel: w153 -> [_ w205]
            tunnel: w154 -> [_ w204]
            tunnel: w156 -> [_ w203]
            tunnel: w160 -> [_ w202]
            tunnel: w159 -> [_ w201]
            tunnel: w158 -> [_ w200]
            tunnel: w157 -> [_ w199]
            tunnel: w170 -> [_ w198]
            tunnel: [w187 w193] -> w169
            tunnel: [w186 w192] -> w168
            tunnel: w167 -> [w187 w197]
            tunnel: w166 -> [w186 w196]
            tunnel: w165 -> [_ w195]
            tunnel: w164 -> [_ w194]
            frame False {
            }
            frame True {
              # "Interpolation"
              n51 = case shown="False" w208 {
                tunnel: w202 -> [w224 w230]
                tunnel: w201 -> [w222 w229]
                tunnel: w200 -> [w221 w228]
                tunnel: w199 -> [w220 w227]
                tunnel: [w223 w226] -> w191
                tunnel: w198 -> [w225 _]
                frame False {
                  n52 = call "IFFT Bin interpolation.vi"("Max Bin"=w224, "Max Amp"=w221, "Prev Max Amp"=w222, "Succ Max Amp"=w220, "Windowing"=w225) -> ("Interpolate Bin"=w223:dbl)
                }
                frame True {
                  n53 = call "Barycentric method RT.vi"("Next Amp"=w227, "Max Bin"=w230, "Max Amp"=w228, "Prev Amp"=w229) -> ("Bin"=w226:dbl)  [unwired: 7 in]
                }
              }
              n54 = case shown="False" w207 {
                tunnel: w206 -> [w210 w219]
                tunnel: w205 -> [w209 w218]
                tunnel: w204 -> [w211 w217]
                tunnel: w203 -> [w213 w216]
                tunnel: [w212 w215] -> w190
                tunnel: w198 -> [w214 _]
                frame False {
                  n55 = call "IFFT Bin interpolation.vi"("Max Bin"=w213, "Max Amp"=w211, "Prev Max Amp"=w210, "Succ Max Amp"=w209, "Windowing"=w214) -> ("Interpolate Bin"=w212:dbl)
                }
                frame True {
                  n56 = call "Barycentric method RT.vi"("Next Amp"=w218, "Max Bin"=w216, "Max Amp"=w217, "Prev Amp"=w219) -> ("Bin"=w215:dbl)  [unwired: 7 in]
                }
              }
              n57 = Divide(x=w191, y=w195) -> (x/y=w189:dbl)
              n58 = Divide(x=w190, y=w194) -> (x/y=w188:dbl)
              n59 = Build Array (concatenate)(w196, w188) -> (w192:dbl[])
              n60 = Build Array (concatenate)(w197, w189) -> (w193:dbl[])
            }
          }
        }
        n61 = case shown="True" w99 {
          tunnel: w108 -> [w120 w126]
          tunnel: [w120 w125] -> w107
          frame False {
          }
          frame True {
            n62 = call <vilib>:"Std Deviation and Variance.vi"("X"=w126) -> ("mean"=w122:dbl, "standard deviation"=w124:dbl)  [unwired: 1 in, 1 out]
            "Distance moving mean" <- w122
            "Mean distance" <- w122
            n63 = Absolute Value(x=w122) -> (abs(x)=w127:dbl)
            n64 = Divide(x=w124, y=w127) -> (x/y=→"Distance moving Rel Standard Deviation" →"Rel Std Dev":dbl)
            n65 = case shown="False" FALSE ("Moving mean") {
              tunnel: w126 -> [_ w132]
              tunnel: [dbl[] [] ("appended array") w129] -> w125
              frame False {
                # "Mean"
              }
              frame True {
                # "Moving mean"
                n66 = Delete From Array(array=w132, length=1, index=0) -> (array with subset deleted=w129:dbl[])  [unwired: 1 out]
              }
            }
          }
        }
        n67 = Array Size(array=w113) -> (size(s)=w111:i32)
        n68 = Greater Than 0?(x=w111) -> (x > 0?=w110:bool)
        n69 = case shown="True" w110 {
          tunnel: w113 -> [_ w147]
          tunnel: w112 -> [_ w146]
          tunnel: w107 -> [w133 w140]
          tunnel: [w133 w139] -> w106
          tunnel: w97 -> [_ w138]
          frame False {
          }
          frame True {
            w148 = 512.0 ("FFT size")
            # "coeff empirico"
            n70 = call <vilib>:"Std Deviation and Variance.vi"("X"=w147) -> ("mean"=w141:dbl)  [unwired: 1 in, 2 out]
            n71 = call <vilib>:"Std Deviation and Variance.vi"("X"=w146) -> ("mean"=w142:dbl)  [unwired: 1 in, 2 out]
            n72 = call "counter 0-N.vi"() -> ("iteration"=w135:fxp<+/-,32,32>)  [unwired: 11 in]
            n73 = Greater Or Equal?(x=w135, y="init scart") -> (x >= y?=w134:bool)
            n74 = call "Frequency from bin number RT.vi"("FFT size"=w148, "Bin number"=w141, "Sample Rate (S/s)"=w138) -> ("Detected Frequency (Hz)"=w145:dbl)  [unwired: 8 in]
            n75 = call "Frequency from bin number RT.vi"("FFT size"=w148, "Bin number"=w142, "Sample Rate (S/s)"=w138) -> ("Detected Frequency (Hz)"=w144:dbl)  [unwired: 8 in]
            n76 = call "Distance-Velocity from Freq.vi"("freq_rising"=w144, "Empirical Distance Costant"=6.201235e-07, "freq_falling"=w145) -> ("Distance (m)"=w137:dbl)  [unwired: 2 in, 2 out]
            n77 = case shown="True" w134 {
              tunnel: w140 -> [w149 w152]
              tunnel: [w149 w151] -> w139
              tunnel: w137 -> [_ w150]
              frame False {
              }
              frame True {
                n78 = Build Array (concatenate)(w152, w150) -> (w151:dbl[])
              }
            }
          }
        }
      }
      frame True {
      }
    }
    n79 = local read "stop"() -> (w84:bool)
    n80 = Select(t=w80, s="Fixed Measure?", f=FALSE ("y")) -> (s? t:f=w79:bool)
    "End" <- w79
    n81 = Or(x=w84, y=w79) -> (x .or. y?=w83:bool)
    n82 = local write "stop"(w79) -> ()
  }
  n83 = while {
    tunnel: w4 -> [w235]
    tunnel: w48 -> [w257]
    tunnel: w21 -> [w254]
    shift-right: [w248] -> w17
    shift-left: w13 -> [w256]
    tunnel: w20 -> [w243]
    tunnel: [w236] -> w16
    tunnel: [w235] -> w15
    stop <- "stop" stop-if-true
    w247 = dbl[] [] ("first subarray")
    w255 = -1 ("Timeout (ms)")
    # "n_signals"
    # "fall+rise"
    # "[Max bin, Max amp, prev amp, next amp] * 2 * 5"
    n84 = xnode "Invoke Method"("FPGA VI Reference In"=w235, "Number of Elements"=w254, "Timeout (ms)"=w255) -> ("Data"=w253:i32[])  [unwired: 1 in, 3 out]
    n85 = xnode "Invoke Method"("FPGA VI Reference In"=w235, "Number of Elements"=w254, "Timeout (ms)"=w255) -> ("Data"=w242:fxp<+,44,44>[])  [unwired: 1 in, 3 out]
    n86 = xnode "Invoke Method"("FPGA VI Reference In"=w235, "Number of Elements"=w254, "Timeout (ms)"=w255) -> ("Data"=w240:fxp<+,44,44>[])  [unwired: 1 in, 3 out]
    n87 = xnode "Invoke Method"("FPGA VI Reference In"=w235, "Number of Elements"=w254, "Timeout (ms)"=w255) -> ("Data"=w238:fxp<+,44,44>[])  [unwired: 1 in, 3 out]
    n88 = for {
      tunnel: w253 -> [w270] mode=indexing
      tunnel: [w269] -> w252 mode=indexing
      n89 = To Double Precision Float(number=w270) -> (double precision float=w269:dbl)
    }
    n90 = To Double Precision Float(number=w240) -> (double precision float=w239:dbl[])
    n91 = To Double Precision Float(number=w238) -> (double precision float=w237:dbl[])
    n92 = To Double Precision Float(number=w242) -> (double precision float=w241:dbl[])
    n93 = Square Root(x=w239) -> (sqrt(x)=w250:dbl[])
    n94 = Square Root(x=w237) -> (sqrt(x)=w249:dbl[])
    n95 = Square Root(x=w241) -> (sqrt(x)=w251:dbl[])
    n96 = Interleave 1D Arrays(w252, w251, w250, w249) -> (w244:dbl[])
    n97 = for {
      N: w243 -> [_]
      shift-right: [w266] -> _
      shift-left: w244 -> [w268]
      shift-right: [w260] -> w246
      shift-left: w247 -> [w261]
      shift-right: [w258] -> w245
      shift-left: w247 -> [w259]
      # "rise"
      # "fall"
      n98 = Split 1D Array(array=w268, index=8) -> (first subarray=w265:dbl[], second subarray=w266:dbl[])
      n99 = Split 1D Array(array=w265, index=4) -> (first subarray=w262:dbl[], second subarray=w263:dbl[])
      n100 = Build Array (concatenate)(w262, w261) -> (w260:dbl[])
      n101 = Build Array (concatenate)(w263, w259) -> (w258:dbl[])
    }
    n102 = Build Array (concatenate)(w246, w245) -> (w234:dbl[])
    n103 = RT FIFO Write(0:w257, 1:w234, 3:w256) -> (8:w236:refnum<k33>, 11:w248:errorcluster)  [unwired: 2 in, 2 out]
  }
  n104 = flat-sequence {
    tunnel: w17 -> [w278]
    tunnel: w15 -> [w273]
    tunnel: w16 -> [w271]
    frame #0 {
      n105 = xnode "Invoke Method"("FPGA VI Reference In"=w273, "error in"=w278) -> ("FPGA VI Reference Out"=w275:refnum<k20>, "error out"=w274:errorcluster)
      n106 = RT FIFO Delete(0:w271) -> ()  [unwired: 2 in, 1 out]
      n107 = property on="stop" class="Bool (strict)"("Value"=FALSE ("stop")) -> ()  [unwired: 2 in, 2 out]
      n108 = xnode "Invoke Method"("FPGA VI Reference In"=w275, "error in"=w274) -> ("FPGA VI Reference Out"=w276:refnum<k20>, "error out"=w277:errorcluster)
      n109 = xnode "Close FPGA VI Reference"("FPGA VI Reference In"=w276, "error in"=w277) -> ()  [unwired: 1 out]
    }
  }
